vi "KE622x -- Turn Output On And Check For Errors.vi"(0 "Resource In":refnum<visa-resource-name>, 1 "Check For SCPI Errors? (T)":bool=TRUE, 5 "Turn Off Output If Compliance?":bool=TRUE, 11 "error in (no error)":errorcluster, 12 "Compliance Check Delay (500 ms)":u32=500) -> (4 "Resource Out (dupl)":refnum<visa-resource-name>, 6 "Interlock Tripped?":bool, 8 "Compliance?":bool, 15 "error out":errorcluster)   [LabVIEW 2025, in "My Current Source.lvlib"]
doc: "Turns on the output of 622x and checks for both a compliance condition or an interlock condition. If the interlock is tripped, the output will not turn on. If the instrument goes into compliance, the user has the option of turning the output off."
uses:
  My Current Source.lvlib
  KE622x -- On Off Control.ctl
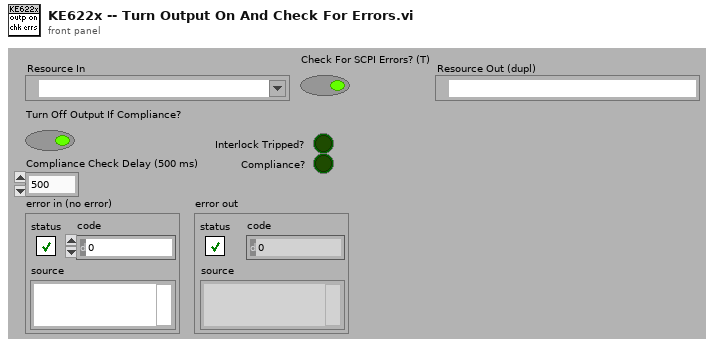
[diagram p1: front panel]
types:
  T1 = typedef "My Current Source.lvlib/KE622x -- On Off Control.ctl" = enum16{"Off", "On"}
  T2 = typedef "My Current Source.lvlib/KE622x -- Meas Event Reg State.ctl" = cluster{"B0, ROF:  KE2182A Delta Reading Overflow Event?":bool, "B1, Int:  Interlock OK Event?":bool, "B2, Temp:  Over Temperature Event?":bool, "B3, Comp:  Compliance Event?":bool, "B5, RAV:  Delta Reading Available Event?":bool, "B6, TN:  User Defined Reading Number Stored In Buffer Event?":bool, "B7, BAV:  At Least 2 Readings Stored In Buffer Event?":bool, "B12, BQF:  Buffer Quarter Full Event?":bool, "B8, BHF:  Buffer Half Full Event?":bool, "B13, B3QF:  Buffer 3/4 Full Event?":bool, "B9, BFL:  Buffer Full Event?":bool}
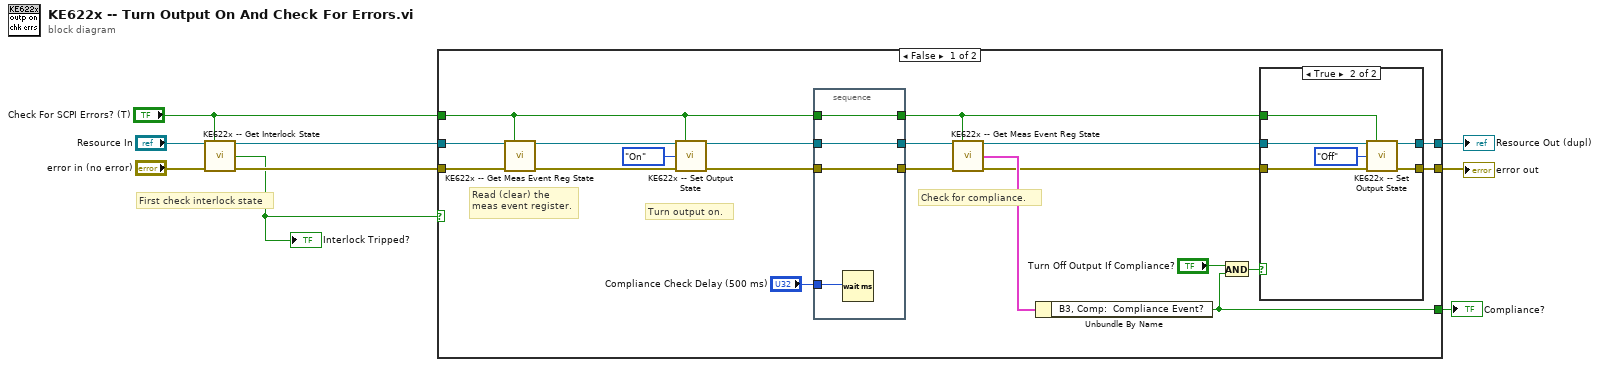
[diagram p0: block diagram]
diagram:
  # "First check interlock state"
  n1 = call "KE622x -- Get Interlock State.vi"("Resource In"="Resource In", "Check For SCPI Errors? (T)"="Check For SCPI Errors? (T)", "error in (no error)"="error in (no error)") -> ("Resource Out (dupl)"=w6:refnum<visa-resource-name>, "Interlock Tripped?"=w4:bool, "error out"=w7:errorcluster)  [unwired: 10 in]
  "Interlock Tripped?" <- w4
  n2 = case shown="False" w4 {
    tunnel: w7 -> [w29 w42]
    tunnel: w6 -> [w28 w43]
    tunnel: "Check For SCPI Errors? (T)" -> [w22 _]
    tunnel: [w16 _] -> w3
    tunnel: [w11 w42] -> w1
    tunnel: [w10 w43] -> w2
    frame False {
      # "Read (clear) the\nmeas event register."
      # "Turn output on."
      # "Check for compliance."
      n3 = call "KE622x -- Get Meas Event Reg State.vi"("VISA Resource In"=w28, "Error Query (T)?"=w22, "error in (no error)"=w29) -> ("VISA Resource Out (dupl)"=w19:refnum<visa-resource-name>, "error out"=w20:errorcluster)  [unwired: 10 in, 1 out]
      n4 = call "KE622x -- Set Output State.vi"("Resource In"=w19, "Check For SCPI Errors? (T)"=w22, "Output State"=KE622x_--_On_Off_Control."On", "error in (no error)"=w20) -> ("Resource Out (dupl)"=w26:refnum<visa-resource-name>, "error out"=w25:errorcluster)  [unwired: 10 in]
      n5 = stacked-sequence {
        tunnel: "Compliance Check Delay (500 ms)" -> [w41]
        tunnel: w26 -> [w40]
        tunnel: w25 -> [w39]
        tunnel: [w40] -> w24
        tunnel: [w39] -> w23
        tunnel: w22 -> [w38]
        tunnel: [w38] -> w12
        frame #0 {
          n6 = Wait (ms)(milliseconds to wait=w41) -> ()  [unwired: 1 out]
        }
      }
      n7 = call "KE622x -- Get Meas Event Reg State.vi"("VISA Resource In"=w24, "Error Query (T)?"=w12, "error in (no error)"=w23) -> ("VISA Resource Out (dupl)"=w14:refnum<visa-resource-name>, "KE622x Meas Event Reg"=w18:T2, "error out"=w13:errorcluster)  [unwired: 10 in]
      n8 = Unbundle By Name(w18) -> ("B3, Comp:  Compliance Event?"=w16:bool)
      n9 = And(x="Turn Off Output If Compliance?", y=w16) -> (x .and. y?=w15:bool)
      n10 = case shown="True" w15 {
        tunnel: w14 -> [w31 w37]
        tunnel: w13 -> [w30 w36]
        tunnel: w12 -> [_ w34]
        tunnel: [w30 w33] -> w11
        tunnel: [w31 w32] -> w10
        frame False {
        }
        frame True {
          n11 = call "KE622x -- Set Output State.vi"("Resource In"=w37, "Check For SCPI Errors? (T)"=w34, "Output State"=KE622x_--_On_Off_Control."Off", "error in (no error)"=w36) -> ("Resource Out (dupl)"=w32:refnum<visa-resource-name>, "error out"=w33:errorcluster)  [unwired: 10 in]
        }
      }
    }
    frame True {
    }
  }
  "Resource Out (dupl)" <- w2
  "error out" <- w1
  "Compliance?" <- w3
